vi "Autonomous Independent.vi"() -> ()   [LabVIEW 2018]
doc: "This VI is called when autonomous begins, and will automatically be terminated when autonomous ends. You can carry out timed or sensor driven robot movement independently without needing to return to the caller."
uses:
  <vilib>/Rock Robotics/WPI/RobotDrive/WPI_RobotDriveDevRef.ctl
  <vilib>/Rock Robotics/WPI/MotorControl/WPI_MotorControlDeviceRef.ctl
  <vilib>/Rock Robotics/WPI/MotorControl/WPI_MotorControlType.ctl
  <vilib>/Rock Robotics/SystemInterfaces/DIO/FPGA_DIOPWMChannel.ctl
  <vilib>/Rock Robotics/WPI/PWM/WPI_PWMDeadband.ctl
  <vilib>/Rock Robotics/SystemInterfaces/DIO/FPGA_DIOChannel.ctl
  <vilib>/Rock Robotics/WPI/Joystick/WPI_JoystickDevRef.ctl
  <vilib>/Rock Robotics/WPI/Joystick/WPI_JoystickDeviceEnum.ctl
  <vilib>/Rock Robotics/WPI/Utilities/WPI_GetSetVariantRefNum.vi
  <vilib>/Rock Robotics/Network Tables/NT Read String.vi
  Robot Global Data.vi
  <vilib>/Rock Robotics/WPI/RobotDrive/WPI_RobotDriveArcadeDrive_Standard(NoSaturation).vi
  <vilib>/Rock Robotics/Network Tables/NT Write Numeric Array.vi
panel:
  out "Current Movement, for debugging":T1 {"Y Joystick Value" scale=1.0..-1.0; "X Joystick Value" scale=-1.0..1.0}
  in  "Array of robot movements":T2(array[cluster])=[{"X Joystick Value"=0.39393939393939403, "Y Joystick Value"=0.0, "Delay (sec)"=1.0, "Movement Name"="turn"}, {"X Joystick Value"=-0.3737373737373737, "Y Joystick Value"=0.0, "Delay (sec)"=1.0, "Movement Name"="turn back"}] {"Y Joystick Value" scale=1.0..-1.0; "X Joystick Value" scale=-1.0..1.0}
  in  "DriveJoystickDevRef":T3
  in  "Drive Motors":T5={"DevStatus"={"status"=FALSE, "code"=0, "source"=""}, "Motors[]"=[], "Square Inputs"=FALSE, "Max Output"=1.0}
  # "Be sure to right-click and choose Data Operations>>Make Current Value default if you want to save the array values with the VI"
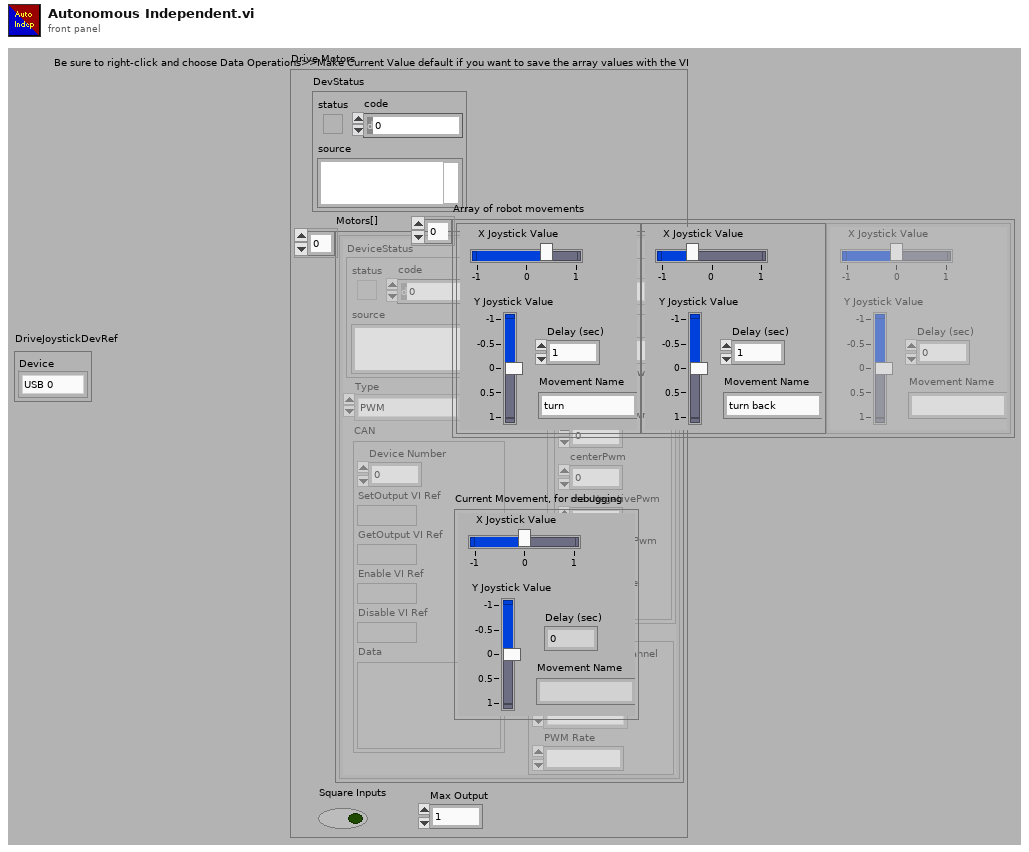
[diagram p1: front panel]
types:
  T1 = cluster{"X Joystick Value":dbl, "Y Joystick Value":dbl, "Delay (sec)":dbl, "Movement Name":string}
  T2 = cluster{"X Joystick Value":dbl, "Y Joystick Value":dbl, "Delay (sec)":dbl, "Movement Name":string}[]
  T3 = typedef "WPI_JoystickDevRef.ctl" = cluster{"Device":T4}
  T4 = typedef "WPI_JoystickDeviceEnum.ctl" = enum16{"USB 0", "USB 1", "USB 2", "USB 3", "USB 4", "USB 5"}
  T5 = typedef "WPI_RobotDriveDevRef.ctl" = cluster{"DevStatus":errorcluster, "Motors[]":T6[], "Square Inputs":bool, "Max Output":dbl}
  T6 = typedef "WPI_MotorControlDeviceRef.ctl" = cluster{"DeviceStatus":errorcluster, "Type":T7, "PWM":cluster{"PWM Channel":T8, "DeadBand":T9}, "CAN":cluster{"Device Number":u8, "SetOutput VI Ref":variant, "GetOutput VI Ref":variant, "Enable VI Ref":variant, "Disable VI Ref":variant, "Data":variant}, "Invert":bool, "DIO PWM":cluster{"PWM \"Enable\" Channel":T8, "DIOChannel":T10, "PWM Rate":dbl}}
  T7 = typedef "WPI_MotorControlType.ctl" = enum16{"PWM", "CAN", "DIO PWM"}
  T8 = typedef "FPGA_DIOPWMChannel.ctl" = enum8{"PWM 0", "PWM 1", "PWM 2", "PWM 3", "PWM 4", "PWM 5", "PWM 6", "PWM 7", "PWM 8", "PWM 9", "PWM MXP 0", "PWM MXP 1", "PWM MXP 2", "PWM MXP 3", "PWM MXP 4", "PWM MXP 5", "PWM MXP 6", "PWM MXP 7", "PWM MXP 8", "PWM MXP 9", "Invalid"}
  T9 = typedef "WPI_PWMDeadband.ctl" = cluster{"Name":string, "maxPositivePwm":i32, "minPositivePwm":i32, "centerPwm":i32, "maxNegativePwm":i32, "minNegativePwm":i32, "angularRange":u16}
  T10 = typedef "FPGA_DIOChannel.ctl" = enum8{"DIO 0", "DIO 1", "DIO 2", "DIO 3", "DIO 4", "DIO 5", "DIO 6", "DIO 7", "DIO 8", "DIO 9", "DIO MXP 0", "DIO MXP 1", "DIO MXP 2", "DIO MXP 3", "DIO MXP 4", "DIO MXP 5", "DIO MXP 6", "DIO MXP 7", "DIO MXP 8", "DIO MXP 9", "DIO MXP 10", "DIO MXP 11", "DIO MXP 12", "DIO MXP 13", "DIO MXP 14", "DIO MXP 15", "SPI Port CS1", "SPI Port CS2", "SPI Port CS3", "SPI Port MISO", "SPI Port MOSI", "Invalid"}
  T11 = cluster{"Drive Motors":T5, "DriveJoystickDevRef":T3}
  T12 = cluster{"Mot Prof Active Velocity":dbl, "Mot Prof Active Position":dbl, "Mot Prof  Is Under Run":bool, "Mot Prof  Has Under Run":bool, "Mot Prof Active Is Last":bool, "Mot Prof Active Is Valid":bool, "Top Mot Prof Count":i32, "Btm Mot Prof Count":i32, "Is Motion Profile Finished?":bool}
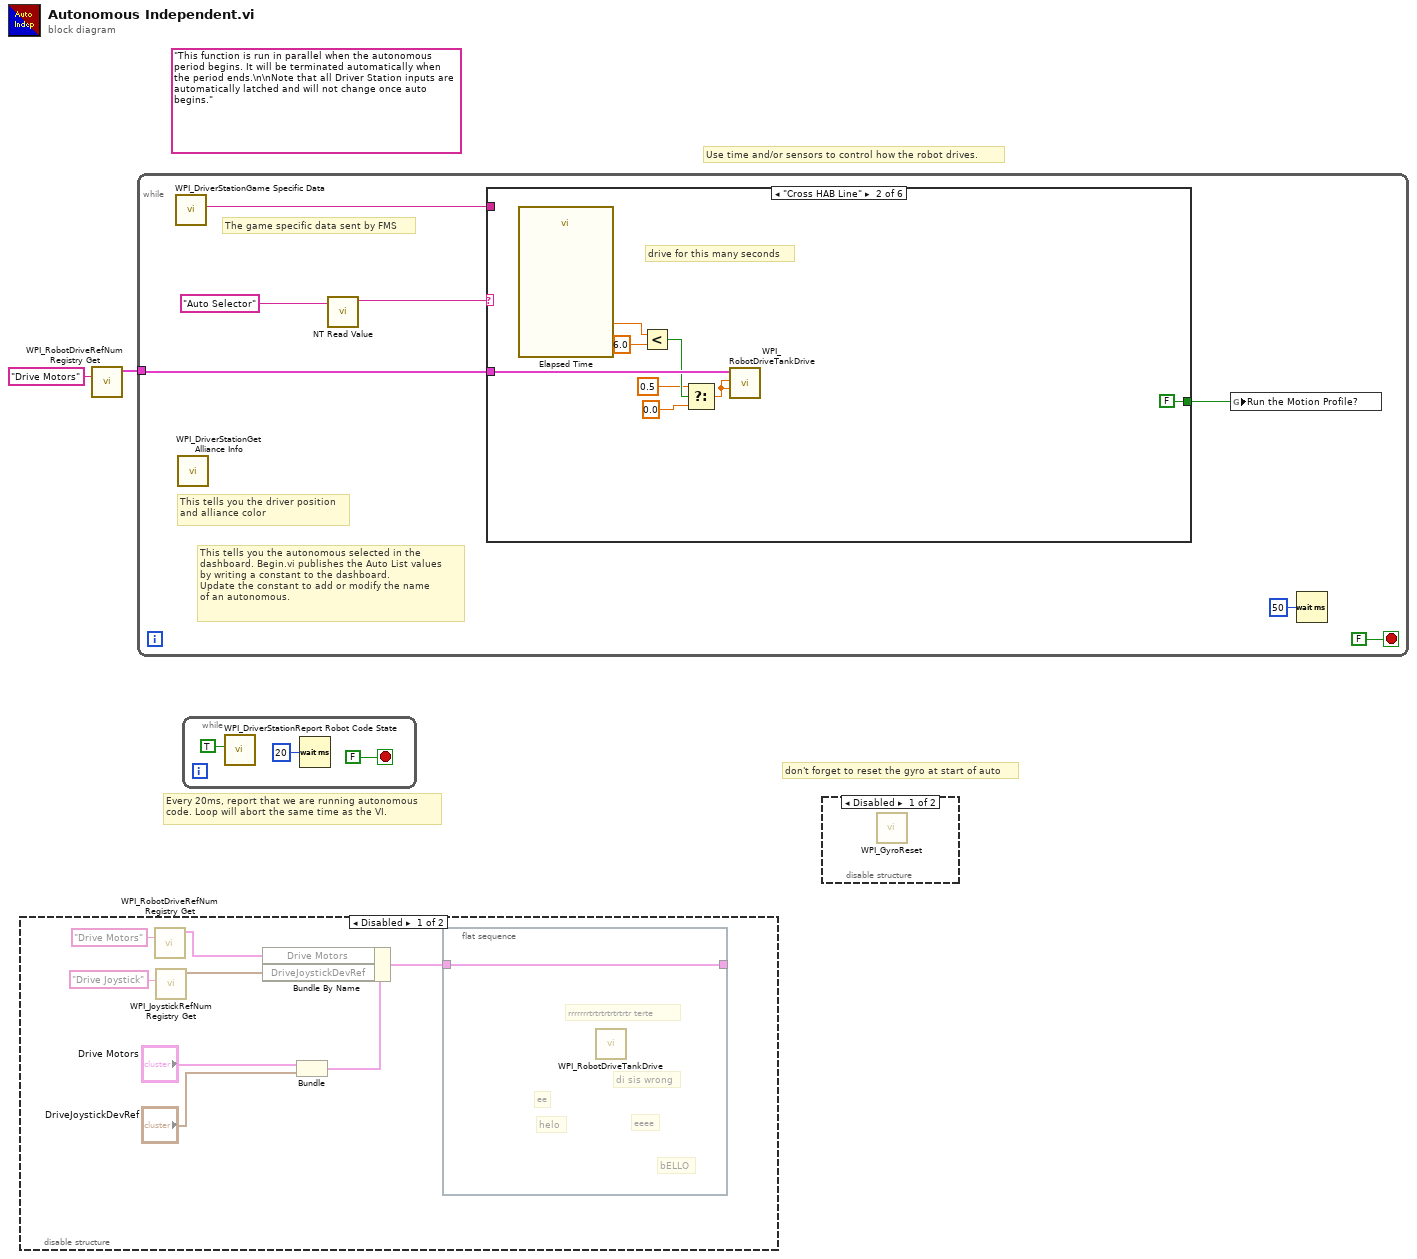
[diagram p0: block diagram]
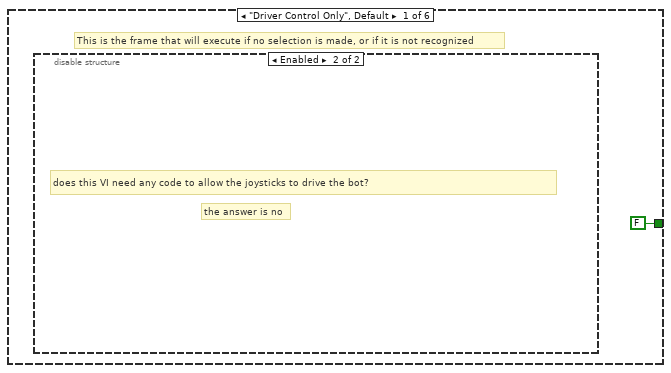
[diagram p2: hidden frame]
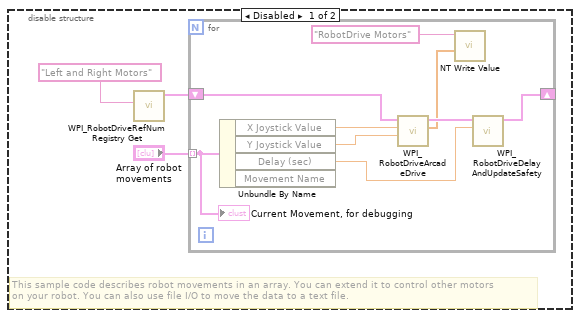
[diagram p3: hidden frame]
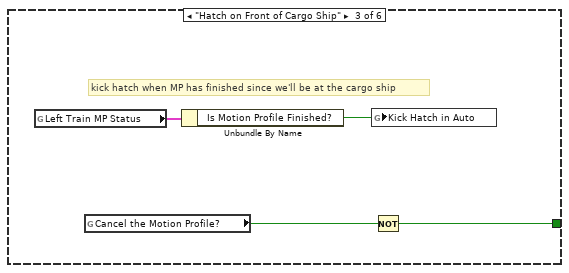
[diagram p4: hidden frame]
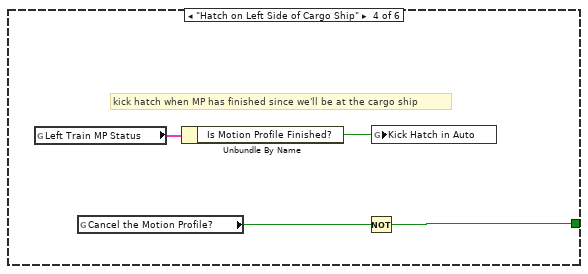
[diagram p5: hidden frame]
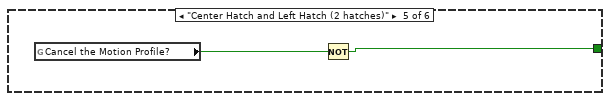
[diagram p6: hidden frame]
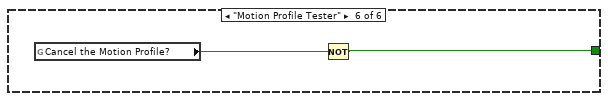
[diagram p7: hidden frame]
diagram:
  (unwired) "This function is run in parallel when the autonomous period begins. It will be terminated automatically when the period ends.\n\nNote that all Driver Station inputs are automatically latched and will not change once auto begins."
  # "don't forget to reset the gyro at start of auto"
  # "Every 20ms, report that we are running autonomous\ncode. Loop will abort the same time as the VI."
  # "Use time and/or sensors to control how the robot drives."
  n1 = disable-structure shown="Disabled" {
    frame Disabled {
      n2 = call <vilib>:"WPI_RobotDriveRefNum Registry Get.vi"("refnum name"="Drive Motors") -> ("RobotDriveDevRef"=w8:T5)  [unwired: 9 in, 1 out]
      n3 = call <vilib>:"WPI_JoystickRefNum Registry Get.vi"("refnum name"="Drive Joystick") -> ("JoystickDevRef"=w7:T3)  [unwired: 9 in, 1 out]
      n4 = Bundle("Drive Motors"="Drive Motors", "DriveJoystickDevRef"="DriveJoystickDevRef") -> (w4:T11)  [unwired: 1 in]
      n5 = Bundle By Name(cluster=w4, "Drive Motors"=w8, "DriveJoystickDevRef"=w7) -> (w3:T11)
      n6 = flat-sequence {
        tunnel: [w11] -> _
        tunnel: w3 -> [w11]
        frame #0 {
          # "eeee"
          # "bELLO"
          # "helo"
          # "ee"
          # "di sis wrong"
          # "rrrrrrrtrtrtrtrtrtrtr terte"
          n7 = call <vilib>:"WPI_RobotDriveTankDrive.vi"() -> ()  [unwired: 9 in, 3 out]
        }
      }
    }
    frame Enabled {
    }
  }
  n8 = call <vilib>:"WPI_RobotDriveRefNum Registry Get.vi"("refnum name"="Drive Motors") -> ("RobotDriveDevRef"=w1:T5)  [unwired: 9 in, 1 out]
  n9 = while {
    tunnel: w1 -> [w12]
    stop <- FALSE stop-if-true
    # "The game specific data sent by FMS"
    # "This tells you the autonomous selected in the \ndashboard. Begin.vi publishes the Auto List values\nby writing a constant to the dashboard.\nUpdate the constant to add or modify the name\nof an autonomous."
    # "This tells you the driver position\nand alliance color"
    n10 = call <vilib>:"WPI_DriverStationGame Specific Data.vi"() -> ("Game Specific Data"=w16:string)  [unwired: 11 in]
    n11 = call <vilib>:"WPI_DriverStationGet Alliance Info.vi"() -> ()  [unwired: 12 out]
    n12 = call-poly <vilib>:"NT Read Value.vi"("Name"="Auto Selector") -> ("String"=w17:string)  [unwired: 9 in, 1 out]
    n13 = case shown="\"Cross HAB Line\"" w17 {
      tunnel: w16 -> [_ _ _ _ _ _]
      tunnel: [FALSE ("Run the Motion Profile?") FALSE ("Run the Motion Profile?") w41 w44 w48 w50] -> w15
      tunnel: w12 -> [_ w38 _ _ _ _]
      frame "Driver Control Only", Default {
        # "This is the frame that will execute if no selection is made, or if it is not recognized"
        n14 = disable-structure shown="Enabled" {
          frame Disabled {
            # "This sample code describes robot movements in an array. You can extend it to control other motors\non your robot. You can also use file I/O to move the data to a text file."
            n15 = call <vilib>:"WPI_RobotDriveRefNum Registry Get.vi"("refnum name"="Left and Right Motors") -> ("RobotDriveDevRef"=w21:T5)  [unwired: 1 in, 9 out]
            n16 = for {
              shift-right: [w29] -> _
              shift-left: w21 -> [w30]
              tunnel: "Array of robot movements" -> [w25] mode=indexing
              n17 = Unbundle By Name(w25) -> ("X Joystick Value"=w28:dbl, "Y Joystick Value"=w27:dbl, "Delay (sec)"=w26:dbl)  [unwired: 1 out]
              n18 = call-poly <vilib>:"WPI_RobotDriveArcadeDrive.vi"("Y axis value"=w27, "X axis value"=w28, "RobotDriveDevRef"=w30) -> ("Motor Values"=w23:dbl[], "RobotDriveDevRef"=w31:T5)  [unwired: 1 in, 6 out]
              n19 = call-poly <vilib>:"NT Write Value.vi"("Numeric Array"=w23, "Name"="RobotDrive Motors") -> ()  [unwired: 9 in, 1 out]
              n20 = call <vilib>:"WPI_RobotDriveDelayAndUpdateSafety.vi"("Delay (s)"=w26, "RobotDriveDevRef"=w31) -> ("RobotDriveDevRef 2"=w29:T5)  [unwired: 8 in, 1 out]
              "Current Movement, for debugging" <- w25
            }
          }
          frame Enabled {
            # "the answer is no"
            # "does this VI need any code to allow the joysticks to drive the bot?"
          }
        }
      }
      frame "Cross HAB Line" {
        # "drive for this many seconds"
        n21 = call "Elapsed Time"() -> ("Elapsed Time (s)"=w37:dbl)  [unwired: 12 in, 7 out]
        n22 = Less?(x=w37, y=6.0) -> (x < y?=w35:bool)
        n23 = Select(t=0.5, s=w35, f=0.0) -> (s? t:f=w32:dbl)
        n24 = call <vilib>:"WPI_RobotDriveTankDrive.vi"("Right axis value"=w32, "Left axis value"=w32, "RobotDriveDevRef"=w38) -> ()  [unwired: 6 in, 3 out]
      }
      frame "Hatch on Front of Cargo Ship" {
        # "kick hatch when MP has finished since we'll be at the cargo ship"
        n25 = global read "Robot Global Data.vi" "Left Train MP Status"() -> (w43:T12)
        n26 = global read "Robot Global Data.vi" "Cancel the Motion Profile?"() -> (w40:bool)
        n27 = Unbundle By Name(w43) -> ("Is Motion Profile Finished?"=w42:bool)
        n28 = global write "Robot Global Data.vi" "Kick Hatch in Auto"(w42) -> ()
        n29 = Not(x=w40) -> (.not. x?=w41:bool)
      }
      frame "Hatch on Left Side of Cargo Ship" {
        # "kick hatch when MP has finished since we'll be at the cargo ship"
        n30 = global read "Robot Global Data.vi" "Left Train MP Status"() -> (w47:T12)
        n31 = global read "Robot Global Data.vi" "Cancel the Motion Profile?"() -> (w45:bool)
        n32 = Unbundle By Name(w47) -> ("Is Motion Profile Finished?"=w46:bool)
        n33 = Not(x=w45) -> (.not. x?=w44:bool)
        n34 = global write "Robot Global Data.vi" "Kick Hatch in Auto"(w46) -> ()
      }
      frame "Center Hatch and Left Hatch (2 hatches)" {
        n35 = global read "Robot Global Data.vi" "Cancel the Motion Profile?"() -> (w49:bool)
        n36 = Not(x=w49) -> (.not. x?=w48:bool)
      }
      frame "Motion Profile Tester" {
        n37 = global read "Robot Global Data.vi" "Cancel the Motion Profile?"() -> (w51:bool)
        n38 = Not(x=w51) -> (.not. x?=w50:bool)
      }
    }
    n39 = global write "Robot Global Data.vi" "Run the Motion Profile?"(w15) -> ()
    n40 = Wait (ms)(milliseconds to wait=u32 50) -> ()  [unwired: 1 out]
  }
  n41 = while {
    stop <- FALSE stop-if-true
    n42 = call <vilib>:"WPI_DriverStationReport Robot Code State.vi"("Autonomous"=TRUE) -> ()  [unwired: 10 in, 1 out]
    n43 = Wait (ms)(milliseconds to wait=u32 20) -> ()  [unwired: 1 out]
  }
  n44 = disable-structure shown="Disabled" {
    frame Disabled {
      n45 = call <vilib>:"WPI_GyroReset.vi"() -> ()  [unwired: 10 in, 2 out]
    }
    frame Enabled {
    }
  }
